vi "saveStateTiming_HEK-v02.vi"(5 "current state":T1=enum."Setting defaults...", 7 "previous state":T1=enum."Setting defaults...", 9 "state times":refnum<vi>, 10 "state list":refnum<vi>, 11 "previous time in":timestamp) -> (3 "previous time out":timestamp)   [LabVIEW 2015]
uses:
  controls/user_message_v6.ctl
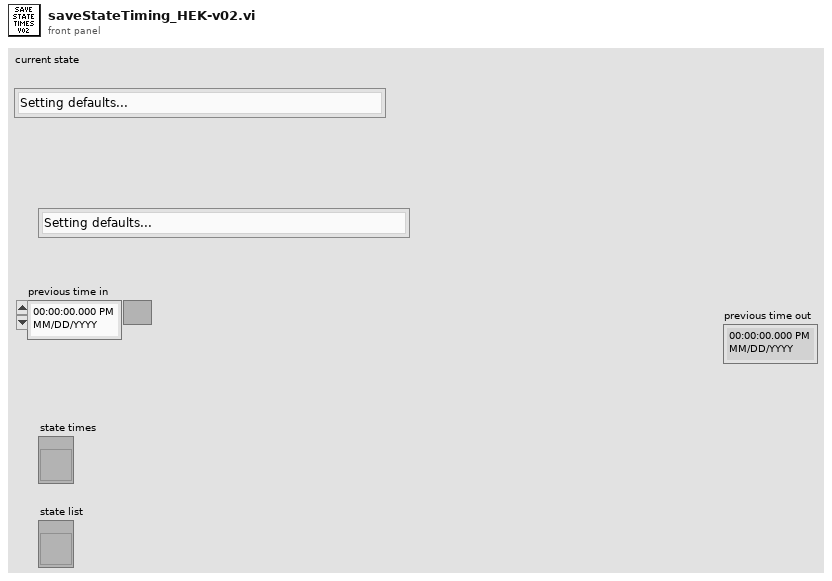
[diagram p1: front panel]
types:
  T1 = typedef "user_message_v6.ctl" = enum16{"Initializing...", "Setting defaults...", "Click OK to start patcherBot!", "Starting new attempt...", "Pipette repositioning...", "Initializing cell tracker...", "Gross approach...", "Human Positioning...", "In Process Calibration", "Detecting cell...", "Cell detected...", "Gigaseal Established...", "Breaking in...", "Successful breakin!", "Unsuccessful breakin!", "Whole-cell recording", "Saving autopatching parameters...", "Quitting VI", "Waiting for idle stage...", "Cleaning...", "Retracting pipette...", "DEBUG STATE", "Waiting to break in...", "Waiting for WC", "reclean", "Done with Current Set of Cells"}
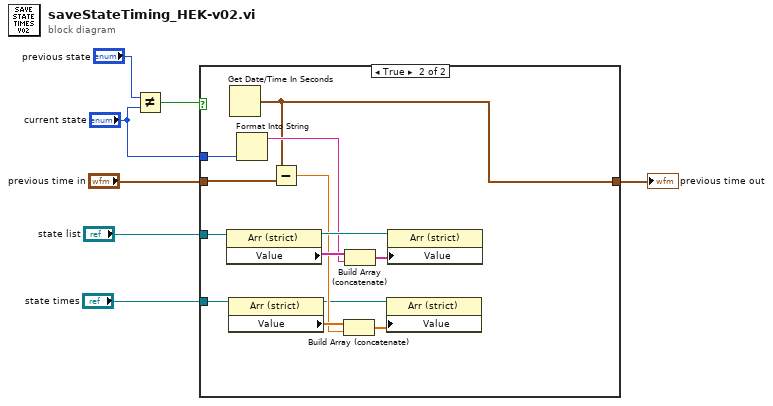
[diagram p0: block diagram]
diagram:
  n1 = Not Equal?(x="previous state", y="current state") -> (x != y?=w7:bool)
  n2 = case shown="True" w7 {
    tunnel: "previous time in" -> [w8 w12]
    tunnel: [w8 w13] -> w5
    tunnel: "current state" -> [_ w21]
    tunnel: "state list" -> [_ w20]
    tunnel: "state times" -> [_ w15]
    frame False {
    }
    frame True {
      n3 = property class="Arr (strict)"(reference=w20) -> (reference out=w19:refnum<vi>, "Value"=w18:string[])  [unwired: 1 in, 1 out]
      n4 = property class="Arr (strict)"(reference=w15) -> (reference out=w10:refnum<vi>, "Value"=w14:dbl[])  [unwired: 1 in, 1 out]
      n5 = Get Date/Time In Seconds() -> (seconds since 1Jan1904=w13:timestamp)
      n6 = Format Into String(w21) -> (resulting string=w17:string)  [unwired: 3 in, 1 out]
      n7 = Subtract(x=w13, y=w12) -> (x-y=w11:dbl)
      n8 = Build Array (concatenate)(w14, w11) -> (w9:dbl[])
      n9 = Build Array (concatenate)(w18, w17) -> (w16:string[])
      n10 = property class="Arr (strict)"(reference=w10, "Value"=w9) -> ()  [unwired: 1 in, 2 out]
      n11 = property class="Arr (strict)"(reference=w19, "Value"=w16) -> ()  [unwired: 1 in, 2 out]
    }
  }
  "previous time out" <- w5
